vi "Pass Channels to Async VIs I32.vi"(11 "Test Case In":refnum<class "Tests Event MessengerM.lvclass">) -> (0 "error out":errorcluster, 3 "Test Case Out":refnum<class "Tests Event MessengerM.lvclass">)   [LabVIEW 2020, in "Tests Event MessengerM.lvclass"]
uses:
  Tests Event MessengerM.lvclass
  C:/Program Files/National Instruments/LabVIEW 2026/vi.lib/Astemes/LUnit/Test Case.lvclass
  <vilib>/Astemes/LUnit/Test Case.lvclass/Test Case.ctl
  <vilib>/Astemes/LUnit/Test Case.lvclass
  b79f69fd-ac2f-4806-84b0-9e56e719c1a6.vi
  ca4d2565-46c2-4d99-81da-89eaa5d06671.vi
  00c4da50-6fd3-4adb-ad10-1b482b76ad5f.vi
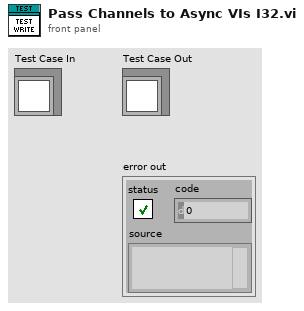
[diagram p1: front panel]
types:
  T1 = typedef "Event MessengerM-i32.lvlib/))Channel.ctl" = refnum<queue>
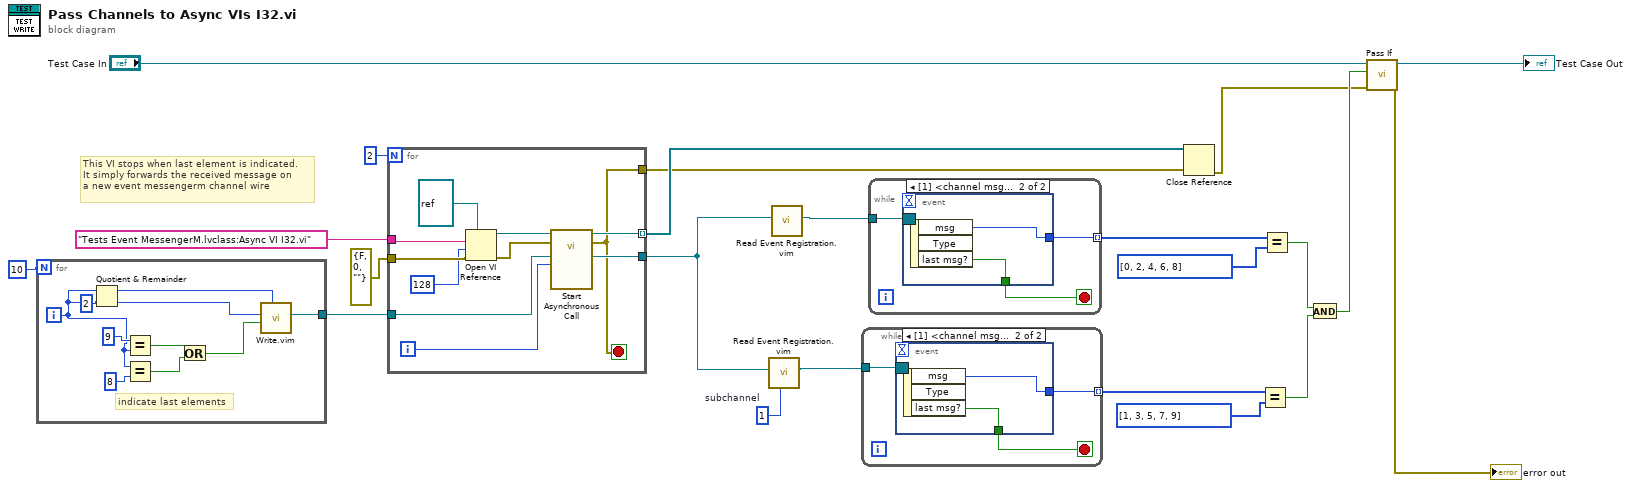
[diagram p0: block diagram]
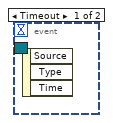
[diagram p2: hidden frame]
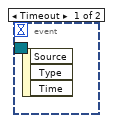
[diagram p3: hidden frame]
diagram:
  w1 = 1  # subchannel
  # "This VI stops when last element is indicated.\nIt simply forwards the received message on\na new event messengerm channel wire"
  n1 = for {
    N: 10 -> [_]
    tunnel: [w25] -> w5
    i -> [w26]
    # "indicate last elements"
    n2 = Quotient & Remainder(x=w26, y=2) -> (x-y*floor(x/y)=w24:i32)  [unwired: 1 out]
    n3 = Equal?(x=9, y=w26) -> (x = y?=w29:bool)
    n4 = Equal?(x=w26, y=8 ("x")) -> (x = y?=w27:bool)
    n5 = Or(x=w29, y=w27) -> (x .or. y?=w23:bool)
    n6 = call "Write.vim"("subchannel"=w24, "last message? (F)"=w23, "element"=w26) -> ("channel"=w25:T1)  [unwired: 7 in, 1 out]
  }
  n7 = for {
    N: 2 -> [_]
    tunnel: "Tests Event MessengerM.lvclass:Async VI I32.vi" -> [w42]
    tunnel: errorcluster {"status"=FALSE, "code"=0, "source"=""} ("error constant") -> [w38]
    tunnel: [w37] -> w2
    tunnel: [w36] -> w8 mode=indexing
    tunnel: [w33] -> w6
    tunnel: w5 -> [w32]
    i -> [w35]
    stop <- w33 stop-if-true
    n8 = Open VI Reference(type specifier VI Refnum (for type only)=refnum<vi> refnum, vi path=w42, options=128, error in (no error)=w38) -> (vi reference=w40:refnum<vi>, error out=w39:errorcluster)  [unwired: 2 in]
    n9 = call-by-ref "Start Asynchronous Call"(reference=w40, error in=w39, "subchannel (0)"=w35, "channel"=w32) -> (reference out=w36:refnum<vi>, error out=w33:errorcluster, "another channel"=w37:T1)  [unwired: 9 in]
  }
  n10 = call "Read Event Registration.vim"("subchannel"=w1, "channel"=w2) -> ("event registration refnum"=w3:refnum<event-registration>)  [unwired: 9 in]
  n11 = call "Read Event Registration.vim"("channel"=w2) -> ("event registration refnum"=w4:refnum<event-registration>)  [unwired: 10 in]
  n12 = while {
    tunnel: w3 -> [w45]
    tunnel: [w44] -> w18 mode=indexing
    stop <- w43 stop-if-true
    n13 = event shown="[1] <channel msg>: User Event" {
      selector: w45 -> [_ _]
      dyn-events: _ -> [_ _]
      timeout: _ -> [_ _]
      tunnel: [_ w47] -> w44
      tunnel: [_ w46] -> w43
      event Timeout {
        n14 = event-data() -> ()  [unwired: 1 in, 3 out]
      }
      event User Event {
        n15 = event-data() -> ("msg"=w47:i32, "last msg?"=w46:bool)  [unwired: 1 in, 1 out]
      }
    }
  }
  n16 = while {
    tunnel: w4 -> [w50]
    tunnel: [w49] -> w15 mode=indexing
    stop <- w48 stop-if-true
    n17 = event shown="[1] <channel msg>: User Event" {
      selector: w50 -> [_ _]
      dyn-events: _ -> [_ _]
      timeout: _ -> [_ _]
      tunnel: [_ w52] -> w49
      tunnel: [_ w51] -> w48
      event Timeout {
        n18 = event-data() -> ()  [unwired: 1 in, 3 out]
      }
      event User Event {
        n19 = event-data() -> ("msg"=w52:i32, "last msg?"=w51:bool)  [unwired: 1 in, 1 out]
      }
    }
  }
  n20 = Close Reference(reference=w8, error in (no error)=w6) -> (error out=w7:errorcluster)
  n21 = Equal?(x=w18, y=i32[] [1, 3, 5, 7, 9] ("Array 2")) -> (x = y?=w16:bool)
  n22 = Equal?(x=w15, y=i32[] [0, 2, 4, 6, 8] ("Array")) -> (x = y?=w13:bool)
  n23 = And(x=w13, y=w16) -> (x .and. y?=w12:bool)
  n24 = call <vilib>:"Pass If.vi"("error in (no error)"=w7, "Pass?"=w12, "LUnit Test Case In"="Test Case In") -> ("error out"=→"error out":errorcluster, "LUnit Test Case Out"=→"Test Case Out":refnum<class "Tests Event MessengerM.lvclass">)  [unwired: 7 in]
